vi "loop timer.vi"(10 "reset":bool, 11 "wait":u32) -> (2 "timing wrong":bool, 3 "loop time out":u32)   [LabVIEW 2018, in "tools.lvlib"]
uses:
  tools.lvlib
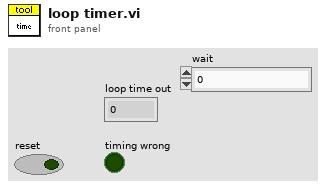
[diagram p1: front panel]
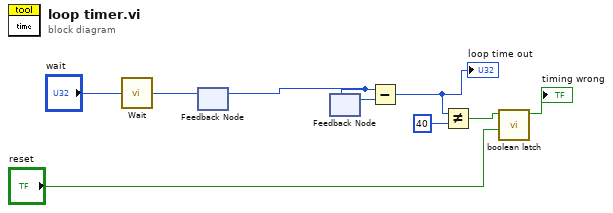
[diagram p0: block diagram]
diagram:
  n1 = call "Wait"("Count(Ticks)"="wait") -> ("Tick Count(Ticks)"=w3:u32)
  n2 = feedback-in #1(w3) -> ()
  n3 = feedback #1() -> (w2:u32)  [unwired: 1 in]
  n4 = feedback #2() -> (w4:u32)  [unwired: 1 in]
  n5 = feedback-in #2(w2) -> ()
  n6 = Subtract(x=w2, y=w4) -> (x-y=w8:u32)
  "loop time out" <- w8
  n7 = Not Equal?(x=w8, y=u32 40) -> (x != y?=w6:bool)
  n8 = call "boolean latch.vi"("clear"="reset", "set"=w6) -> ("out"=→"timing wrong":bool)  [unwired: 9 in]
